vi "Autoscale Multi-XY as Needed_modded.vi"(1 "axis attributes":T1={"x minimum"=0.0, "x maximum"=0.0, "x log?"=FALSE, "x precision"=1, "x format"=enum."Decimal", "y minimum"=0.0, "y maximum"=0.0, "y log?"=FALSE, "y precision"=1, "y format"=enum."Decimal"} {"x minimum" format="%0.2f"; "x maximum" format="%0.2f"; "y minimum" format="%0.2f"; "y maximum" format="%0.2f"}, 2 "multi-xy data":cluster{"data":cluster{"x":dbl, "y":dbl}[]}[](array[cluster]) {"data"."y" format="%0.2f"; "data"."x" format="%0.2f"}) -> (0 "axis attributes":T1={"x minimum"=0.0, "x maximum"=0.0, "x log?"=FALSE, "x precision"=1, "x format"=enum."Decimal", "y minimum"=0.0, "y maximum"=0.0, "y log?"=FALSE, "y precision"=1, "y format"=enum."Decimal"} {"x minimum" format="%0.2f"; "x maximum" format="%0.2f"; "y minimum" format="%0.2f"; "y maximum" format="%0.2f"})   [LabVIEW 2018]
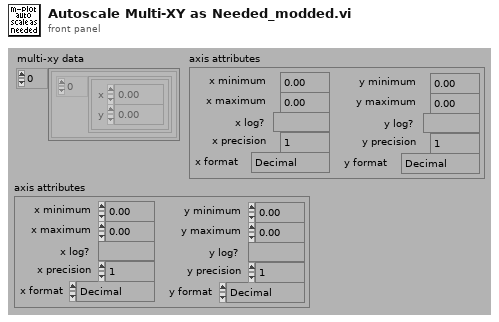
[diagram p1: front panel]
types:
  T1 = cluster{"x minimum":dbl, "x maximum":dbl, "x log?":bool, "x precision":u8, "x format":enum8{"Decimal", "Scientific", "Engineering", "Binary", "Octal", "Hex", "Timestamp"}, "y minimum":dbl, "y maximum":dbl, "y log?":bool, "y precision":u8, "y format":enum8{"Decimal", "Scientific", "Engineering", "Binary", "Octal", "Hex", "Timestamp"}}
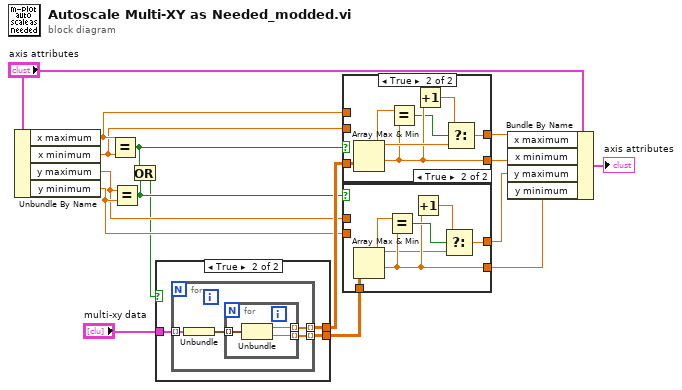
[diagram p0: block diagram]
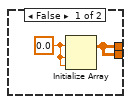
[diagram p2: hidden frame]
diagram:
  n1 = Unbundle By Name("axis attributes") -> ("x maximum"=w15:dbl, "x minimum"=w14:dbl, "y maximum"=w12:dbl, "y minimum"=w13:dbl)
  n2 = Equal?(x=w15, y=w14) -> (x = y?=w10:bool)
  n3 = Equal?(x=w12, y=w13) -> (x = y?=w9:bool)
  n4 = Or(x=w10, y=w9) -> (x .or. y?=w8:bool)
  n5 = case shown="True" w8 {
    tunnel: "multi-xy data" -> [_ w21]
    tunnel: [w17 w20] -> w16
    tunnel: [w17 w19] -> w7
    frame False {
      w18 = 0.0
      n6 = Initialize Array(w18, w18, w18) -> (w17:dbl[][])
    }
    frame True {
      n7 = for {
        tunnel: w21 -> [w25] mode=indexing
        tunnel: [w23] -> w20 mode=indexing
        tunnel: [w22] -> w19 mode=indexing
        n8 = Unbundle(w25) -> ("data"=w24:cluster{"x":dbl, "y":dbl}[])
        n9 = for {
          tunnel: w24 -> [w28] mode=indexing
          tunnel: [w27] -> w23 mode=indexing
          tunnel: [w26] -> w22 mode=indexing
          n10 = Unbundle(w28) -> ("x"=w27:dbl, "y"=w26:dbl)
        }
      }
    }
  }
  n11 = case shown="True" w10 {
    tunnel: w15 -> [w29 _]
    tunnel: w14 -> [w30 _]
    tunnel: [w30 w35] -> w11
    tunnel: w16 -> [_ w31]
    tunnel: [w29 w33] -> w6
    frame False {
    }
    frame True {
      n12 = Array Max & Min(array=w31) -> (max value=w36:dbl, min value=w35:dbl)  [unwired: 2 out]
      n13 = Equal?(x=w36, y=w35) -> (x = y?=w34:bool)
      n14 = Increment(x=w35) -> (x+1=w32:dbl)
      n15 = Select(t=w32, s=w34, f=w36) -> (s? t:f=w33:dbl)
    }
  }
  n16 = case shown="True" w9 {
    tunnel: w13 -> [w37 _]
    tunnel: w12 -> [w38 _]
    tunnel: w7 -> [_ w44]
    tunnel: [w37 w40] -> w4
    tunnel: [w38 w42] -> w5
    frame False {
    }
    frame True {
      n17 = Array Max & Min(array=w44) -> (max value=w39:dbl, min value=w40:dbl)  [unwired: 2 out]
      n18 = Equal?(x=w39, y=w40) -> (x = y?=w41:bool)
      n19 = Increment(x=w40) -> (x+1=w43:dbl)
      n20 = Select(t=w43, s=w41, f=w39) -> (s? t:f=w42:dbl)
    }
  }
  n21 = Bundle By Name(cluster="axis attributes", "x maximum"=w6, "x minimum"=w11, "y maximum"=w5, "y minimum"=w4) -> (→"axis attributes":T1)
